vi "Read Multi Eval Meas Spectrum Average Results.vi"(8 "error in (no error)":errorcluster, 10 "Instance (1)":i32=1, 11 "VISA resource name":refnum<visa-resource-name>) -> (0 "error out":errorcluster, 1 "Out Of Tolerance":dbl format="%^.3e", 2 "Reliability":i32, 3 "VISA resource name out":refnum<visa-resource-name>, 4 "Results":dbl[](array[numeric]) format="%^.3e")   [LabVIEW 2020, in "Rohde&Schwarz CMP LR WPAN Measurement.lvlib"]
doc: "Starts a new single shot measurement and returns the average spectrum results. Returns string of 22 single values.\n\nAttribute:\n-\n\nRemote-control command:\nREAD:WPAN:MEAS<i>:MEValuation:SPECtrum:AVERage?"
uses:
  <instrlib>/Rohde&Schwarz CMP LR WPAN Measurement/Rohde&Schwarz CMP LR WPAN Measurement.lvlib
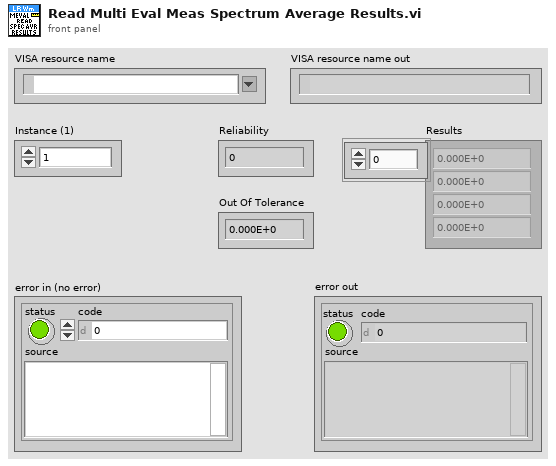
[diagram p1: front panel]
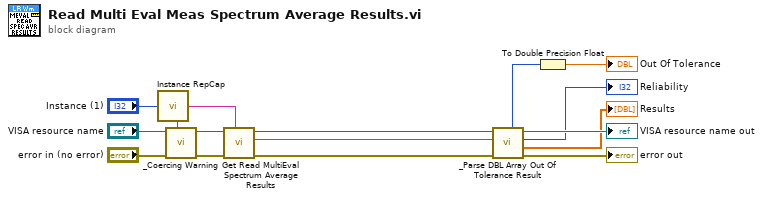
[diagram p0: block diagram]
diagram:
  n1 = call <instrlib>:"Instance RepCap.vi"("Instance In"="Instance (1)") -> ("In Range?"=w15:bool, "RepCap Identifier Out"=w16:string)  [unwired: 1 in]
  n2 = call <instrlib>:"_Coercing Warning.vi"("In Range?"=w15, "error in (no error)"="error in (no error)", "VISA resource name"="VISA resource name") -> ("error out"=w12:errorcluster, "VISA resource name out"=w11:refnum<visa-resource-name>)  [unwired: 7 in]
  n3 = call "Get Read MultiEval Spectrum Average Results"("Repeated Capabilities"=w16, "error in (no error)"=w12, "instrument handle"=w11) -> ("error out"=w9:errorcluster, "Read MultiEval Spectrum Average Results"=w8:string, "instrument handle out"=w10:refnum<visa-resource-name>)  [unwired: 6 in]
  n4 = call <instrlib>:"_Parse DBL Array Out Of Tolerance Result.vi"("error in (no error)"=w9, "Input String"=w8, "VISA resource name"=w10) -> ("error out"=→"error out":errorcluster, "Results"=→"Results":dbl[], "Reliability"=→"Reliability":i32, "VISA resource name out"=→"VISA resource name out":refnum<visa-resource-name>, "Out Of Tolerance"=w7:i32)  [unwired: 4 in]
  n5 = To Double Precision Float(number=w7) -> (double precision float=→"Out Of Tolerance":dbl)
